vi "aula6 1.vi"() -> ()   [LabVIEW 2026]
uses:
  <vilib>/Instr/_visa.llb/VISA Configure Serial Port (Instr).vi
panel:
  in  "Boolean 2":bool
  in  "Boolean":bool
  out "read buffer":string
  in  "byte count":u32
  in  "Enable Termination\nChar (T)":bool=TRUE
  in  "stop bits (10: 1 bit)":u16(ring)=10 items=["1.0"=10, "1.5"=15, "2.0"=20]
  in  "parity (0:none)":enum16{"None", "Odd", "Even", "Mark", "Space"}(ring)
  in  "data bits (8)":u16=8 min=5 max=8 step=1
  in  "baud rate (9600)":u32=9600
  in  "stop 3":bool
  in  "stop 2":bool
  in  "stop":bool
  in  "termination char\n(0xA = '\\n' = LF)":u8=10 format="%.0x"
  in  "VISA resource name":refnum<visa-resource-name>
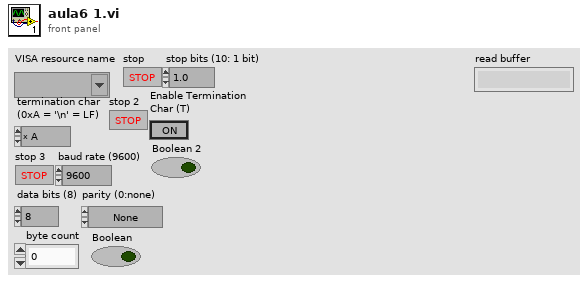
[diagram p1: front panel]
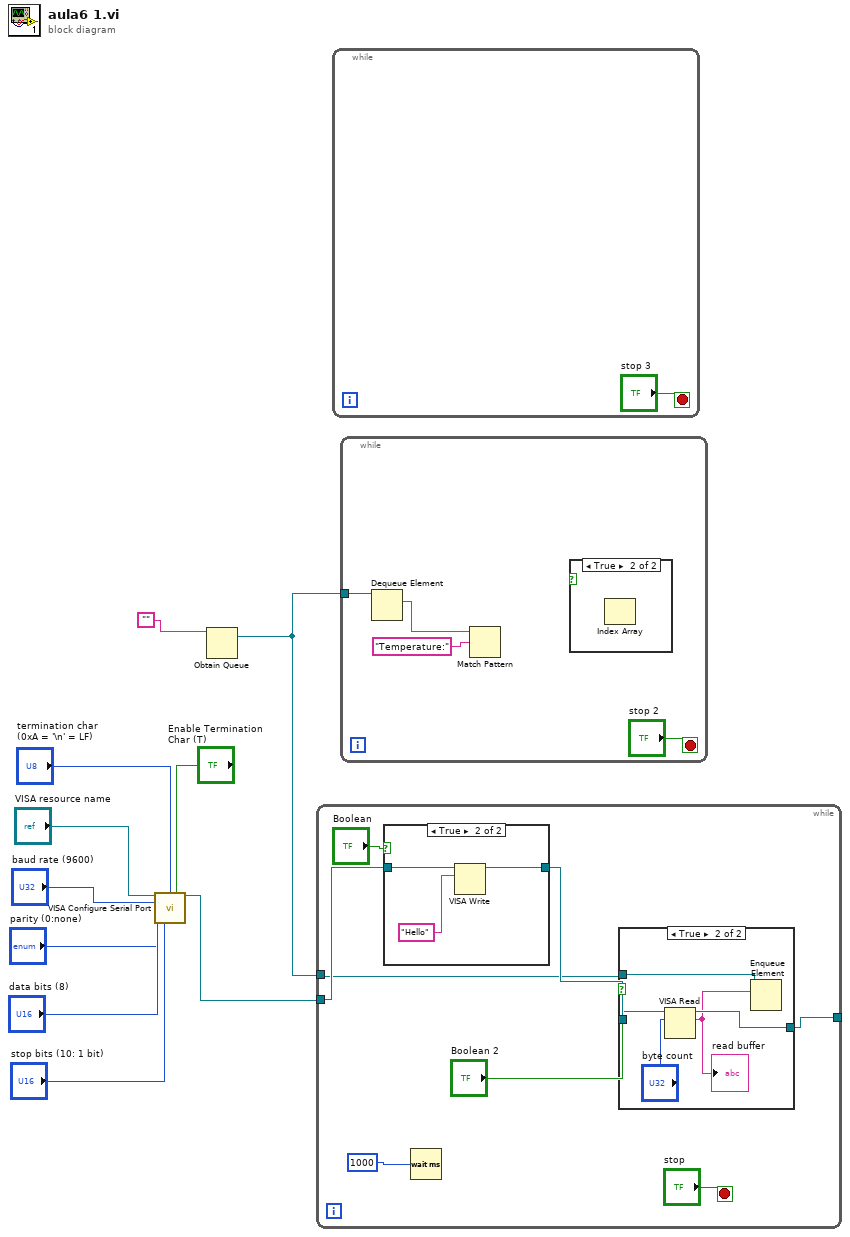
[diagram p0: block diagram]
diagram:
  n1 = call-poly "VISA Configure Serial Port"("VISA resource name"="VISA resource name", "termination char\n(0xA = '\\n' = LF)"="termination char\n(0xA = '\\n' = LF)", "Enable Termination\nChar (T)"="Enable Termination\nChar (T)", "baud rate (9600)"="baud rate (9600)", "data bits (8)"="data bits (8)", "parity (0:none)"="parity (0:none)", "stop bits (10: 1 bit)"="stop bits (10: 1 bit)") -> ("VISA resource name out"=w8:refnum<visa-resource-name>)  [unwired: 7 in, 1 out]
  n2 = Obtain Queue(name (unnamed)="") -> (queue out=w1:refnum<queue>)  [unwired: 4 in, 2 out]
  n3 = while {
    tunnel: w8 -> [w16]
    tunnel: [w12] -> _
    tunnel: w1 -> [w11]
    stop <- "stop" stop-if-true
    n4 = case shown="True" "Boolean" {
      tunnel: w16 -> [w25 w28]
      tunnel: [w25 w26] -> w14
      frame False {
      }
      frame True {
        n5 = VISA Write(VISA resource name=w28, write buffer="Hello") -> (VISA resource name out=w26:refnum<visa-resource-name>)  [unwired: 1 in, 2 out]
      }
    }
    n6 = Wait (ms)(milliseconds to wait=u32 1000) -> ()  [unwired: 1 out]
    n7 = case shown="True" "Boolean 2" {
      tunnel: w14 -> [w19 w24]
      tunnel: [w19 w22] -> w12
      tunnel: w11 -> [_ w20]
      frame False {
      }
      frame True {
        n8 = VISA Read(VISA resource name=w24, byte count="byte count") -> (VISA resource name out=w22:refnum<visa-resource-name>, read buffer=w21:string)  [unwired: 1 in, 2 out]
        "read buffer" <- w21
        n9 = Enqueue Element(queue=w20, element=w21) -> ()  [unwired: 2 in, 3 out]
      }
    }
  }
  n10 = while {
    stop <- "stop 3" stop-if-true
  }
  n11 = while {
    tunnel: w1 -> [w30]
    stop <- "stop 2" stop-if-true
    n12 = Dequeue Element(queue=w30) -> (element=w32:string)  [unwired: 2 in, 3 out]
    n13 = Match Pattern(string=w32, regular expression="Temperature:") -> ()  [unwired: 1 in, 4 out]
    n14 = case shown="True" {
      selector: _ -> [_ _]
      frame False {
      }
      frame True {
        n15 = Index Array() -> ()  [unwired: 2 in, 1 out]
      }
    }
  }
